vi "o3 Serial Data Recording & DECADEv3.1_test.vi"() -> ()   [LabVIEW 2014]
uses:
  <vilib>/Platform/TimedLoop/XDataNode/timing_clust.ctl
  <vilib>/Platform/TimedLoop/XDataNode/nitl_modes.ctl
  <vilib>/Platform/TimedLoop/XDataNode/wakeup.ctl
  C:/Program Files (x86)/National Instruments/LabVIEW 2014/examples/Data Communication/Network Streams/Simple Network Streams/support/Network Stream Command.ctl
  <vilib>/Utility/error.llb/whitespace.ctl
  <vilib>/Instr/_visa.llb/VISA Configure Serial Port (Instr).vi
  <vilib>/Utility/tcp.llb/UDP Multicast Write-Only Open.vi
  <vilib>/platform/TimedLoop/XDataNode/XDataNode.xnode
  <vilib>/Platform/TimedLoop/XDataNode/XDNodeRunTimeDep.lvlib
panel:
  out "Stop File Write":bool
  out "Default file name":string
  out "error out":errorcluster
  out "V6":bool
  in  "Clear Display\nErrors":bool
  out "Data Processing":bool
  out "Serial Visa Error":errorcluster
  out "SEPTIC TCP Error Out":errorcluster
  out "TCP packet\nSend to SEPTIC":bool
  in  "Time Stamp\nOffset":u32=1
  out "Data Array":string[](array[string])
  out "UDP packet \nstatus":bool
  out "UDP_Out_Error":errorcluster
  out "FISH TCP Error Out":errorcluster
  out "TCP packet\nSend to FISH":bool
  out "TCP Binary Packet":string
  out "Scan from String Error Counter\nfrom process loop":i32
  out "Read Error Counter\nfrom process loop":i32
  in  "milliseconds to wait":u32=330
  in  "ID":string="±"
  in  "VISA resource name":refnum<visa-resource-name>="ASRL6::INSTR"
  out "Data In Array":string[](array[string])
  out "UDP_ASCII_Out":string
  out "UDP_Pack_num":u32
  out "Flight Number":string
  in  "aux":string="0"
  in  "inlet_overq_mfm":string="0"
  in  "acs2653pc_hdd":string="0"
  in  "LabviewVIclient vn":string="0"
  in  "ue9LJ temp":u16
  in  "PTP Sync":string="0"
  out "Data String":string
  out "Internal packet":string[](array[string])
  out "RAW DATA":string
  in  "stop":bool
  out "Number of Send & Read Error\nfrom Acquire Loop":i32
  out "Command In":string
  # "o3_conc"
  # "Bench_temp"
  # "pressure"
  # "cell_a_nt"
  # "cell_b_int"
  # "flow_a"
  # "flow_b"
  # "lamp_temp"
  # "flags"
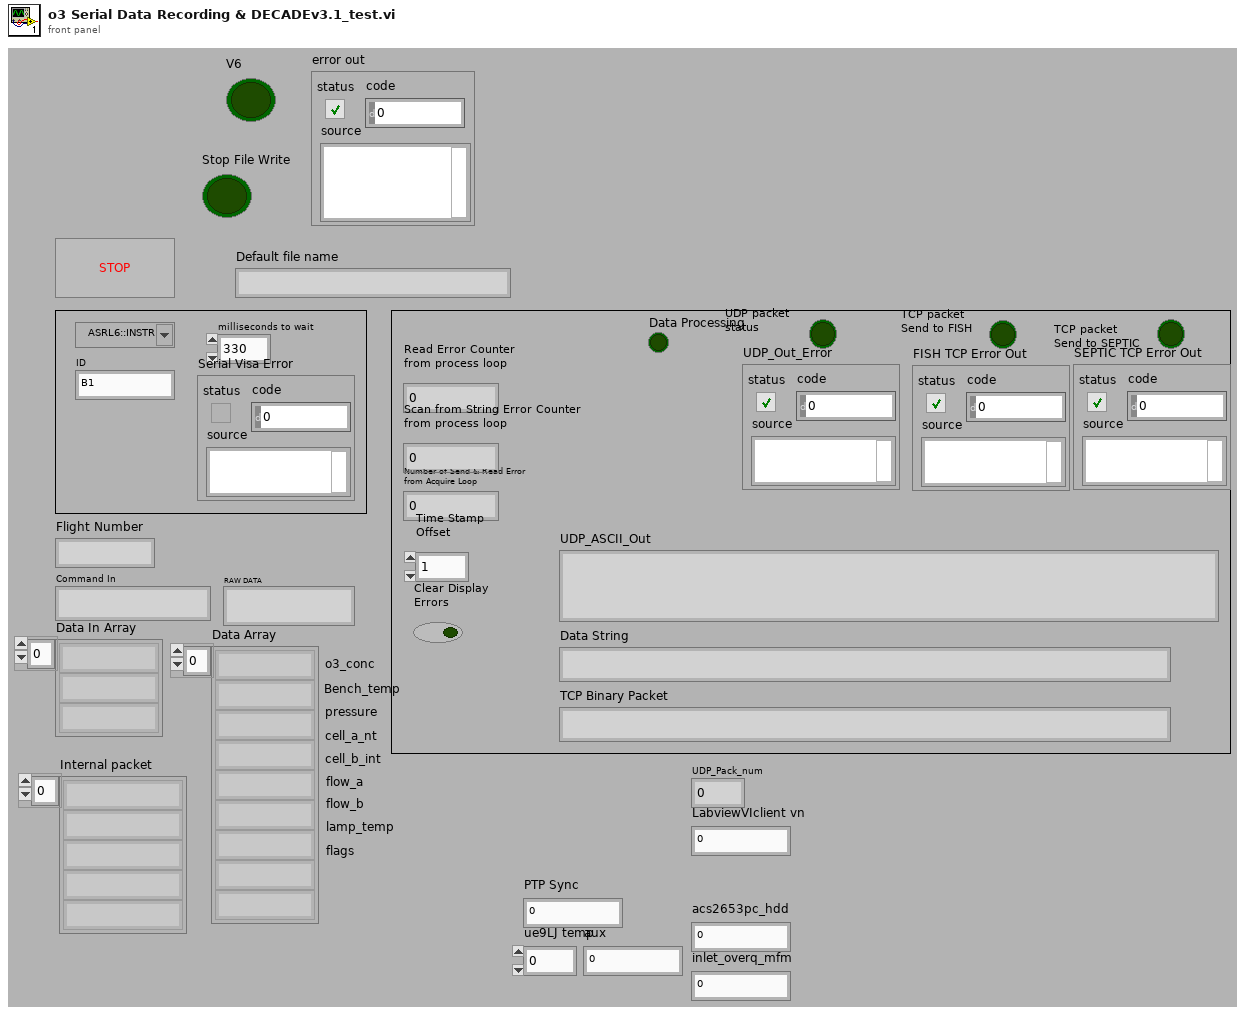
[diagram p1: front panel]
types:
  T1 = typedef "XDNodeRunTimeDep.lvlib/timing_clust.ctl" = cluster{"Expected End [f-1]":u64, "Actual End [f-1]":u64, "Finished Late? [f-1]":bool, "Expected End [i-1]":u64, "Actual End [i-1]":u64, "Finished Late? [i-1]":bool, "Expected Start [i]":u64, "Actual Start [i]":u64, "Expected Start [f]":u64, "Actual Start [f]":u64, "Source Name":string, "Structure Name":string, "Period":i64, "Deadline":i64, "Offset":i64, "Start":i64, "Priority":i32, "Timeout":i32, "Mode":T2, "Wakeup Reason":T3, "Error":errorcluster, "Source Type":string, "Secondary Source Type":string, "Global End Time":u64, "Global Start Time":u64, "Frame Duration":u64, "Iteration Duration":u64, "Assigned CPU":i32, "I/O Scan Engine Mode":u32}
  T2 = typedef "XDNodeRunTimeDep.lvlib/nitl_modes.ctl" = enum32{"No Change", "Process missed periods, maintain original phase", "Discard missed periods, maintain original phase", "Process missed periods, ignore original phase", "Discard missed periods, ignore original phase"}
  T3 = typedef "XDNodeRunTimeDep.lvlib/wakeup.ctl" = enum32{"Normal", "Aborted", "Asynchronous wakeup", "Timing source error", "Timed loop error", "Timeout"}
  T4 = typedef "Network Stream Command.ctl" = cluster{"Message":string, "Message Data":variant}
  T5 = enum16{"open", "replace", "create", "open or create", "replace or create", "replace or create with confirmation"}
  T6 = typedef "whitespace.ctl" = u16
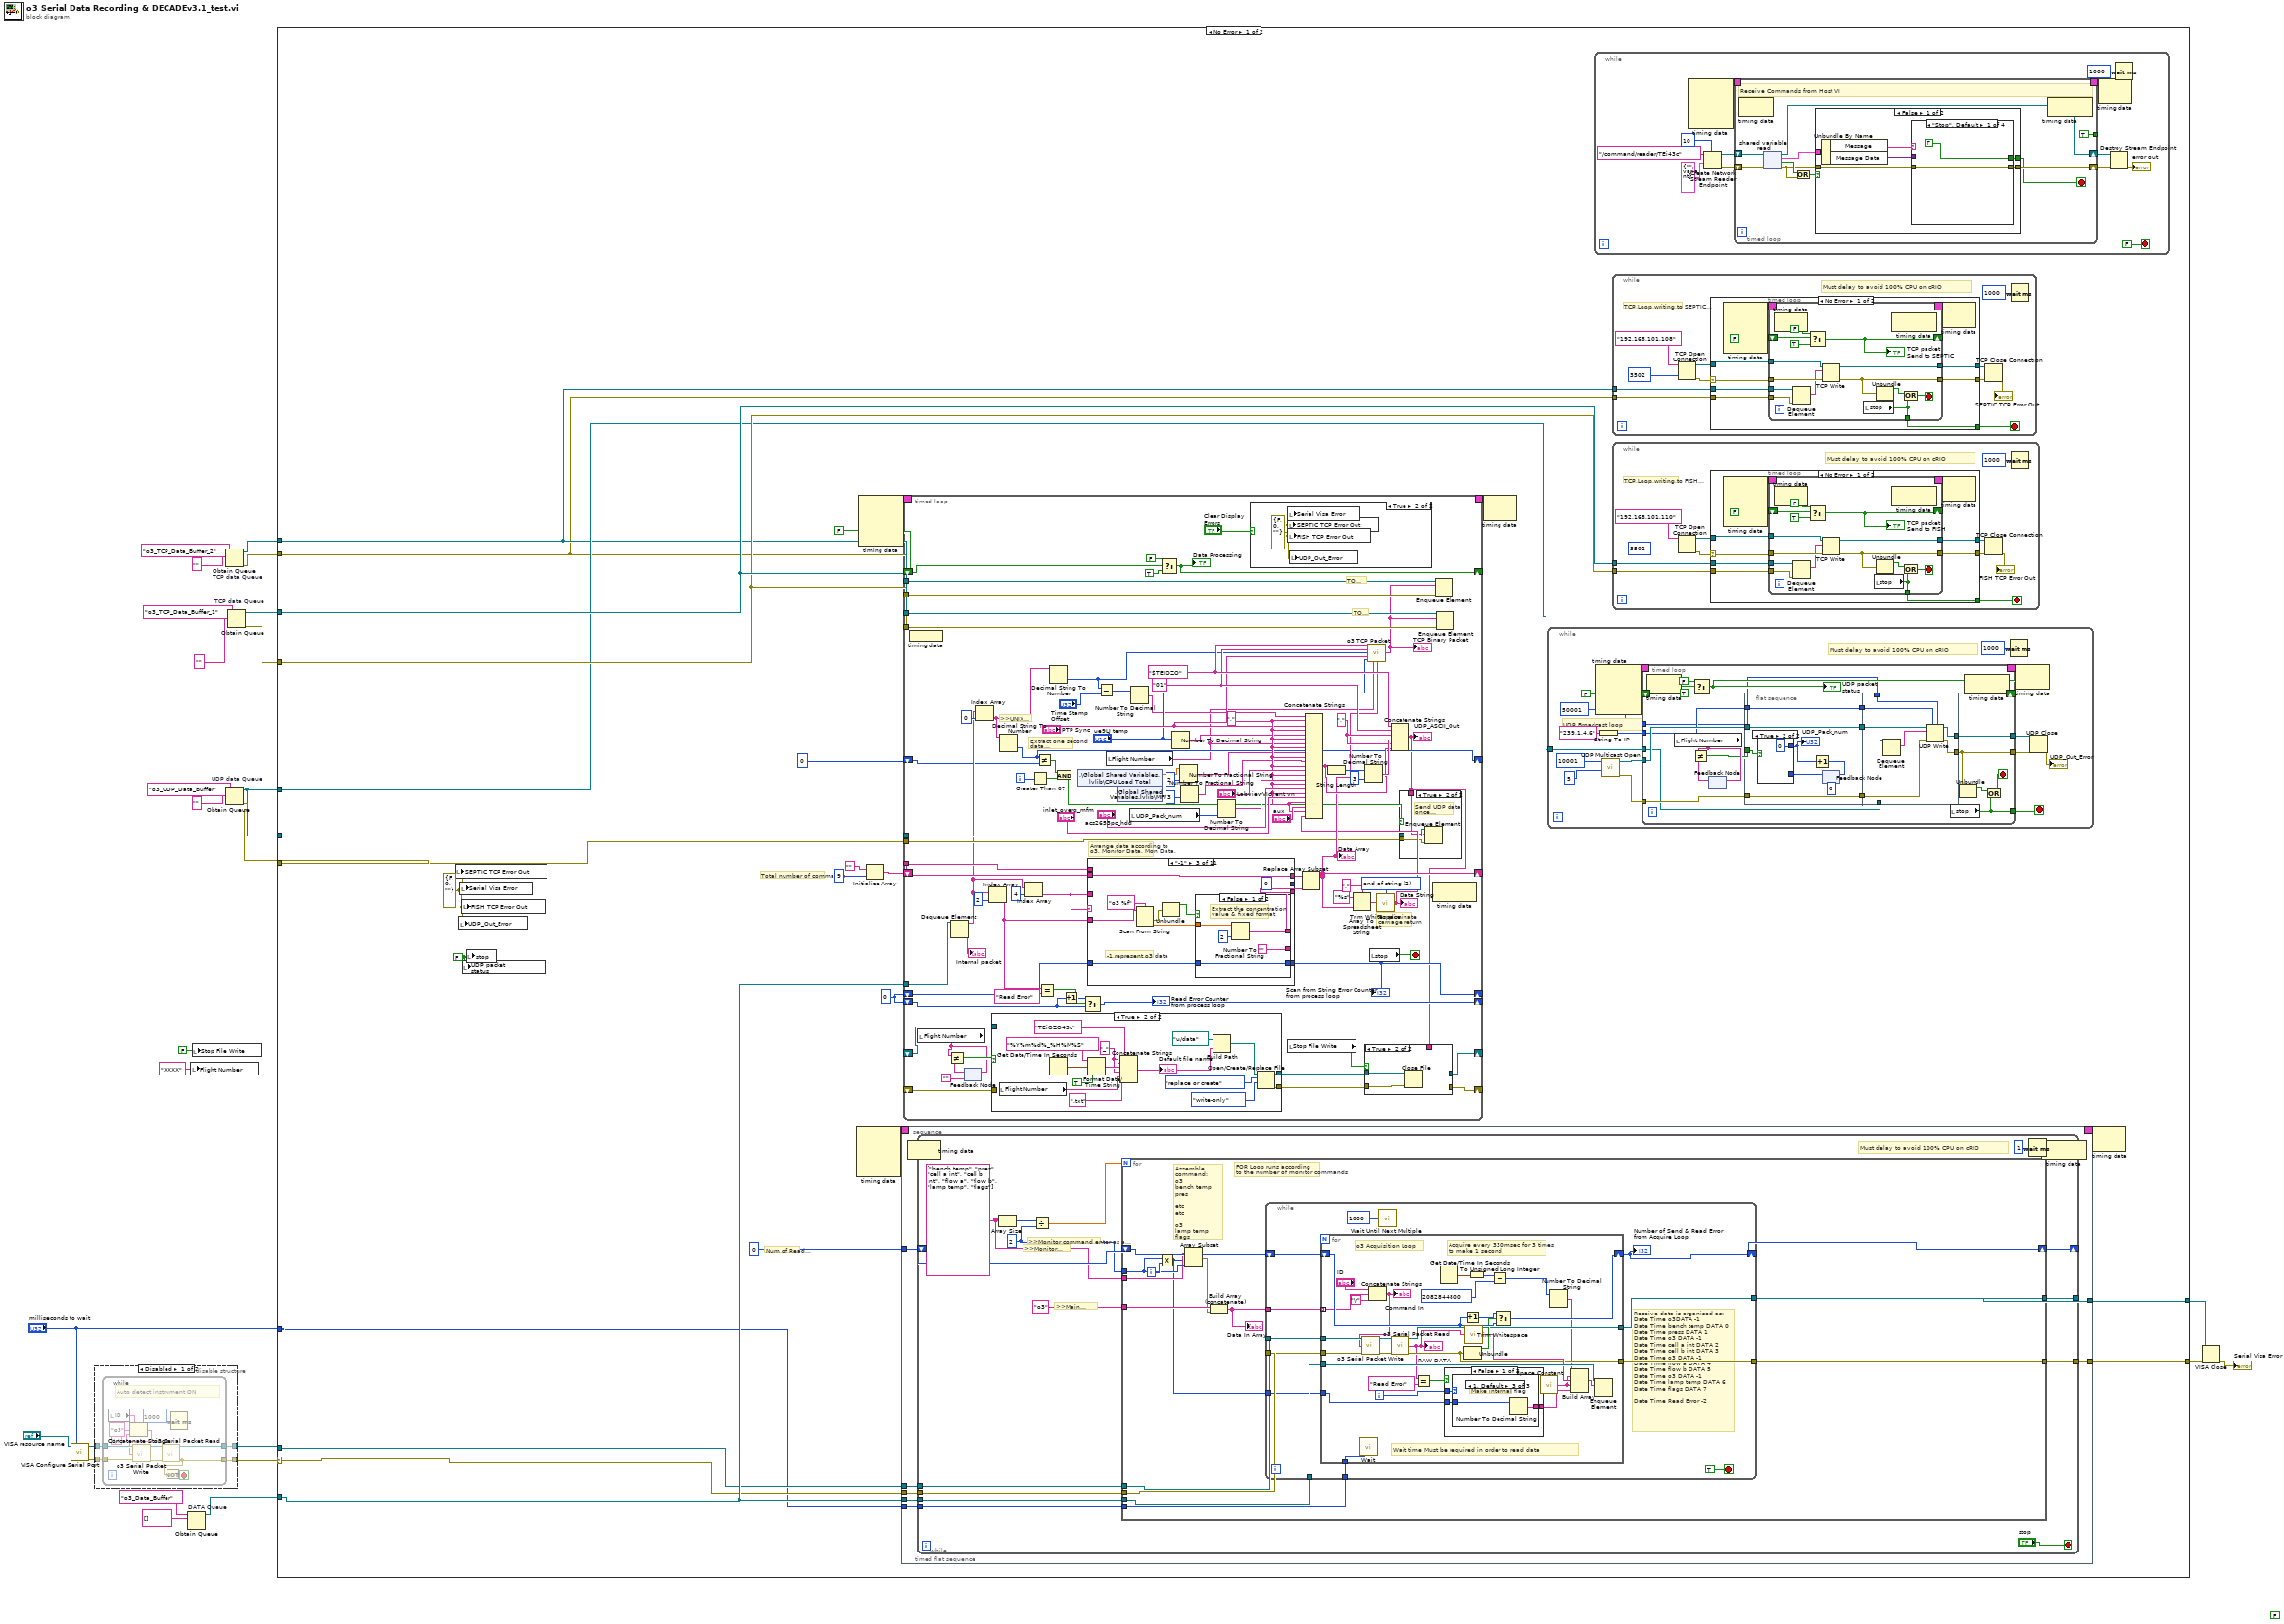
[diagram p0: block diagram]
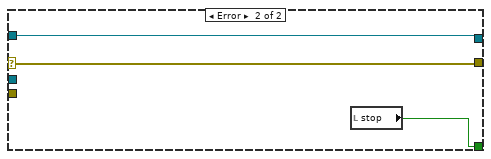
[diagram p3: hidden frame]
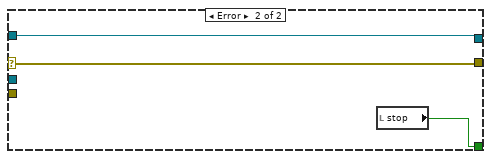
[diagram p4: hidden frame]
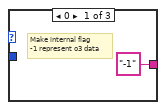
[diagram p5: hidden frame]
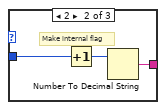
[diagram p6: hidden frame]
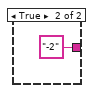
[diagram p7: hidden frame]
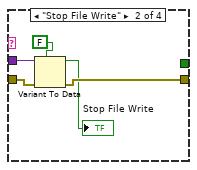
[diagram p8: hidden frame]
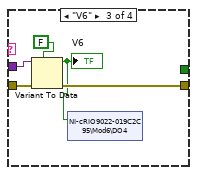
[diagram p9: hidden frame]
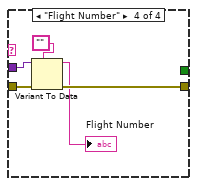
[diagram p10: hidden frame]
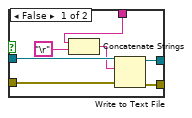
[diagram p14: hidden frame]
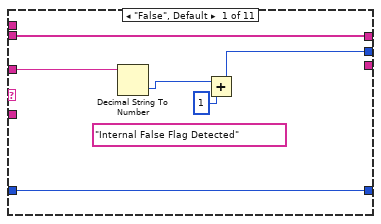
[diagram p17: hidden frame]
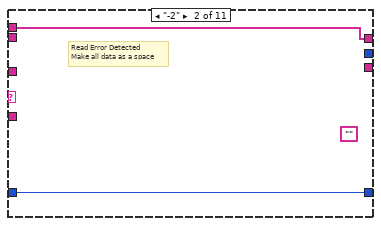
[diagram p18: hidden frame]
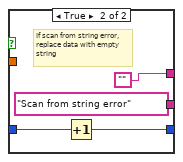
[diagram p19: hidden frame]
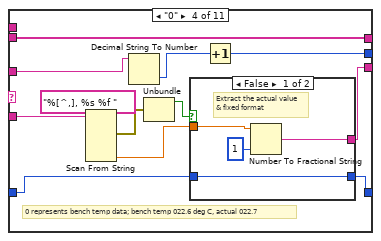
[diagram p20: hidden frame]
diagram:
  (unwired) FALSE
  n1 = call-poly "VISA Configure Serial Port"("VISA resource name"="VISA resource name", "timeout (10sec)"="milliseconds to wait") -> ("VISA resource name out"=w8:refnum<visa-resource-name>, "error out"=w7:errorcluster)  [unwired: 12 in]
  n2 = disable-structure shown="Disabled" {
    disable-tunnel: [w30 _] -> w10
    disable-tunnel: [w29 _] -> w9
    disable-tunnel: w8 -> [w28 _]
    disable-tunnel: w7 -> [w27 _]
    frame Disabled {
      n3 = while {
        tunnel: [w40] -> w30
        tunnel: [w39] -> w29
        tunnel: w28 -> [w38]
        tunnel: w27 -> [w37]
        stop <- w41 stop-if-true
        # "Auto detect instrument ON"
        n4 = local read "ID"() -> (w35:string)
        n5 = Concatenate Strings(w35, "o3" ("string"), "\r") -> (w32:string)
        n6 = call "o3 Serial Packet Write.vi"("VISA resource name In"=w38, "Data in"=w32, "error in (no error)"=w37) -> ("VISA resource name Out"=w36:refnum<visa-resource-name>, "error out"=w42:errorcluster)  [unwired: 11 in]
        n7 = call "o3 Serial Packet Read.vi"("VISA resource In"=w36, "error in"=w42) -> ("VISA resource Out"=w39:refnum<visa-resource-name>, "error out"=w40:errorcluster)  [unwired: 11 in, 1 out]
        n8 = Not(x=w40) -> (.not. x?=w41:bool)
        n9 = Wait (ms)(milliseconds to wait=u32 1000) -> ()  [unwired: 1 out]
      }
    }
    frame Enabled {
    }
  }
  n10 = Obtain Queue "DATA Queue"(name (unnamed)="o3_Data_Buffer", element data type=string[] []) -> (queue out=w24:refnum<queue>)  [unwired: 3 in, 2 out]
  n11 = local write "Flight Number"("XXXX" ("Flight Number")) -> ()
  n12 = local write "Stop File Write"(FALSE ("Stop File Write")) -> ()
  n13 = Obtain Queue "TCP data Queue"(name (unnamed)="o3_TCP_Data_Buffer_2", element data type="") -> (queue out=w13:refnum<queue>, error out=w12:errorcluster)  [unwired: 3 in, 1 out]
  n14 = Obtain Queue "UDP data Queue"(name (unnamed)="o3_UDP_Data_Buffer", element data type="") -> (queue out=w14:refnum<queue>, error out=w15:errorcluster)  [unwired: 3 in, 1 out]
  n15 = Obtain Queue "TCP data Queue"(name (unnamed)="o3_TCP_Data_Buffer_1", element data type="") -> (queue out=w19:refnum<queue>, error out=w18:errorcluster)  [unwired: 3 in, 1 out]
  n16 = case shown="No Error" w10 {
    selector: w10 -> [w52 w673]
    tunnel: [w68 w673] -> w21
    tunnel: [w67 w672] -> w22
    tunnel: w24 -> [w64 _]
    tunnel: w9 -> [w51 w672]
    tunnel: w19 -> [w57 _]
    tunnel: w18 -> [w56 _]
    tunnel: w14 -> [w55 _]
    tunnel: w15 -> [w54 _]
    tunnel: w14 -> [w53 _]
    tunnel: w13 -> [w49 _]
    tunnel: w12 -> [w48 _]
    tunnel: "milliseconds to wait" -> [w47 _]
    frame No Error {
      w45 = errorcluster {"status"=FALSE, "code"=0, "source"=""} ("UDP Error Out")
      w59 = 0
      w58 = FALSE ("stop")
      # "Num of Read Error"
      # "Total number of commands"
      n17 = local write "SEPTIC TCP Error Out"(w45) -> ()
      n18 = local write "UDP_Out_Error"(w45) -> ()
      n19 = local write "Serial Visa Error"(w45) -> ()
      n20 = local write "FISH TCP Error Out"(w45) -> ()
      n21 = local write "UDP packet \nstatus"(w58) -> ()
      n22 = local write "stop"(w58) -> ()
      n23 = node-c288() -> (w44:T1)  [unwired: 4 in]
      n24 = node-c288() -> (w66:T1)  [unwired: 4 in]
      n25 = Initialize Array("", 9) -> (w60:string[])
      n26 = timed-sequence {
        timing: w44 -> [_]
        timing-out: [_] -> w43
        tunnel: [w159] -> w68
        tunnel: [w158] -> w67
        tunnel: w64 -> [w157]
        tunnel: 0 -> [w156]
        tunnel: w52 -> [w155]
        tunnel: w51 -> [w154]
        tunnel: w47 -> [w153]
        n27 = timed-flat-sequence {
          tunnel: [w166] -> w159
          tunnel: [w165] -> w158
          tunnel: w157 -> [w164]
          tunnel: w156 -> [w163]
          tunnel: w155 -> [w162]
          tunnel: w154 -> [w161]
          tunnel: w153 -> [w160]
          n28 = node-c288() -> ()  [unwired: 1 in, 1 out]
          n29 = while {
            tunnel: [w170] -> w166
            tunnel: w161 -> [w181]
            tunnel: w162 -> [w180]
            tunnel: [w179] -> w165
            tunnel: w164 -> [w178]
            shift-right: [w176] -> _
            shift-left: w163 -> [w177]
            tunnel: w160 -> [w168]
            stop <- "stop" stop-if-true
            w171 = 2
            w173 = string[] ["bench temp", "pres", "cell a int", "cell b int", "flow a", "flow b", "lamp temp", "flags"]
            # "Must delay to avoid 100% CPU on cRIO"
            # ">>Monitor command enter as a pair>>"
            # ">>Main commands>>"
            # ">>Monitor Command>>"
            n30 = Array Size(array=w173) -> (size(s)=w174:i32)
            n31 = Divide(x=w174, y=w171) -> (x/y=w172:dbl)
            n32 = for {
              N: w172 -> [_]
              tunnel: w181 -> [w189]
              tunnel: w180 -> [w188]
              tunnel: [w196] -> w170
              shift-right: [w194] -> w176
              shift-left: w177 -> [w195]
              tunnel: [w193] -> w179
              tunnel: w178 -> [w192]
              tunnel: w173 -> [w185]
              tunnel: "o3" -> [w190]
              tunnel: w171 -> [w186]
              tunnel: w168 -> [w182]
              i -> [w187]
              # "FOR Loop runs according\nto the number of monitor commands"
              # "Assemble command:\no3\nbench temp\npres\n\netc\netc\n\no3\nlamp temp\nflags"
              n33 = Multiply(x=w186, y=w187) -> (x*y=w183:i32)
              n34 = Array Subset(array=w185, index=w183, length=w186) -> (w184:string[])
              n35 = Build Array (concatenate)(w190, w184) -> (w191:string[])
              "Data In Array" <- w191
              n36 = while {
                tunnel: [w208] -> w196
                tunnel: w191 -> [w206]
                tunnel: [w204] -> w193
                tunnel: w192 -> [w203]
                tunnel: w188 -> [w202]
                tunnel: w189 -> [w201]
                tunnel: w183 -> [w200]
                shift-right: [w205] -> w194
                shift-left: w195 -> [w207]
                tunnel: w182 -> [w197]
                stop <- TRUE stop-if-true
                # "Receive data is organised as:\nDate Time o3DATA -1\nDate Time bench temp DATA 0\nDate Time press DATA 1\nDate Time o3 DATA -1\nDate Time cell a int DATA 2\nDate Time cell b int DATA 3\nDate Time o3 DATA -1\nDate Time flow a DATA 4\nDate Time flow b DATA 5\nDate Time o3 DATA -1\nDate Time lamp temp DATA 6\nDate Time flags DATA 7\n\nDate Time Read Error -2"
                n37 = for {
                  tunnel: w202 -> [w225]
                  tunnel: [w226] -> w208
                  tunnel: w206 -> [w223] mode=indexing
                  tunnel: [w227] -> w204
                  tunnel: w203 -> [w233]
                  tunnel: w201 -> [w228]
                  tunnel: w200 -> [w222]
                  shift-right: [w237] -> w205
                  shift-left: w207 -> [w238]
                  tunnel: w197 -> [w211]
                  i -> [w215]
                  # "Wait time Must be required in order to read data"
                  # "Acquire every 330msec for 3 times\nto make 1 second"
                  # "o3 Acquisition Loop"
                  n38 = call "Wait"("Count(mSec)"=w211) -> ()  [unwired: 1 out]
                  n39 = Concatenate Strings("ID", w223, "\r") -> (w221:string)
                  "Command In" <- w221
                  n40 = call "o3 Serial Packet Write.vi"("VISA resource name In"=w228, "Data in"=w221, "error in (no error)"=w225) -> ("VISA resource name Out"=w230:refnum<visa-resource-name>, "error out"=w229:errorcluster)  [unwired: 11 in]
                  n41 = call "o3 Serial Packet Read.vi"("VISA resource In"=w230, "error in"=w229) -> ("VISA resource Out"=w227:refnum<visa-resource-name>, "Data Out"=w218:string, "error out"=w226:errorcluster)  [unwired: 11 in]
                  "RAW DATA" <- w218
                  n42 = Equal?(x=w218, y="Read Error") -> (x = y?=w216:bool)
                  n43 = Get Date/Time In Seconds() -> (seconds since 1Jan1904=w210:timestamp)
                  n44 = case shown="False" w216 {
                    tunnel: [w241 "-2"] -> w231
                    tunnel: w215 -> [w240 _]
                    tunnel: w222 -> [w239 _]
                    frame False {
                      n45 = case shown="1, Default" w240 {
                        tunnel: ["-1" w245 w247] -> w241
                        tunnel: w239 -> [_ w243 w246]
                        frame 0 {
                          # "Make internal flag\n-1 represent o3 data"
                        }
                        frame 2 {
                          # "Make internal flag"
                          n46 = Increment(x=w243) -> (x+1=w244:i32)
                          n47 = Number To Decimal String(number=w244) -> (decimal integer string=w245:string)  [unwired: 1 in]
                        }
                        frame 1, Default {
                          # "Make internal flag"
                          n48 = Number To Decimal String(number=w246) -> (decimal integer string=w247:string)  [unwired: 1 in]
                        }
                      }
                    }
                    frame True {
                    }
                  }
                  n49 = Increment(x=w238) -> (x+1=w234:i32)
                  n50 = Unbundle(w226) -> ("status"=w235:bool)  [unwired: 2 out]
                  n51 = call <vilib>:"Trim Whitespace.vi"("string"=w218) -> ("trimmed string"=w232:string)  [unwired: 1 in]
                  n52 = To Unsigned Long Integer(number=w210) -> (unsigned 32bit integer=w214:u32)
                  n53 = Subtract(x=w214, y=u32 2082844800) -> (x-y=w209:u32)
                  n54 = Select(t=w234, s=w235, f=w238) -> (s? t:f=w237:i32)
                  n55 = call <vilib>:"Space Constant.vi"() -> ("String"=w219:string)
                  n56 = Number To Decimal String(number=w209) -> (decimal integer string=w212:string)  [unwired: 1 in]
                  n57 = Build Array(w212, w219, w232, w219, w231) -> (w220:string[])
                  n58 = Enqueue Element(queue=w233, element=w220) -> ()  [unwired: 2 in, 3 out]
                }
                "Number of Send & Read Error\nfrom Acquire Loop" <- w205
                n59 = call "Wait Until Next Multiple"("Count(mSec)"=u32 1000) -> ()  [unwired: 1 out]
              }
            }
            n60 = Wait (ms)(milliseconds to wait=u32 1) -> ()  [unwired: 1 out]
          }
          n61 = node-c288() -> ()  [unwired: 1 in, 1 out]
        }
      }
      n62 = timed-loop {
        timing: w66 -> [_]
        timing-out: [_] -> w65
        tunnel: w64 -> [w446]
        shift-right: [w407] -> _
        shift-left: w60 -> [w430]
        shift-right: [w418] -> _
        shift-left: w59 -> [w415]
        tunnel: w60 -> [w417]
        shift-right: [w413] -> _
        shift-left: w59 -> [w414]
        tunnel: w57 -> [w406]
        tunnel: w56 -> [w405]
        tunnel: w55 -> [w403]
        tunnel: w54 -> [w402]
        shift-right: [w394] -> _
        shift-left: 0 -> [w397]
        tunnel: w49 -> [w392]
        tunnel: w48 -> [w391]
        shift-right: [w382] -> _
        shift-left: FALSE -> [w385]
        shift-right: [w379] -> _
        shift-left: _ -> [w370]
        shift-right: [w368] -> _
        shift-left: _ -> [w369]
        i -> [w395]
        stop <- w444 stop-if-true
        w423 = T6 2 items=["both", "start of string", "end of string"] ("location (both)")
        w436 = ","
        w410 = "01"
        w432 = ","
        w411 = "$TEIOZO"
        # "TO SEPTIC"
        # "TO FISH"
        # "Extract one second data\nfor UDP sending"
        # "Arrange data according to\no3, Monitor Data, Mon Data,"
        # "To eliminate\ncarriage return"
        # ">>UNIX TIME>>"
        n63 = node-c288() -> ()  [unwired: 1 in]
        n64 = local read "Flight Number"() -> (w373:string)
        n65 = Dequeue Element(queue=w446) -> (element=w400:string[])  [unwired: 2 in, 3 out]
        "Internal packet" <- w400
        n66 = feedback #1("" ("Flight Number")) -> (w375:string)
        n67 = Not Equal?(x=w373, y=w375) -> (x != y?=w374:bool)
        n68 = feedback-in #1(w373) -> ()
        n69 = Index Array(array=w400, index=0) -> (element=w399:string)
        n70 = Index Array(array=w400, index=2) -> (element=w421:string)
        n71 = case shown="True" w374 {
          tunnel: [w448 w450] -> w372
          tunnel: [w447 w449] -> w371
          tunnel: w370 -> [w448 _]
          tunnel: w369 -> [w447 _]
          frame False {
          }
          frame True {
            w457 = "_" ("string")
            n72 = local read "Flight Number"() -> (w463:string)
            n73 = Get Date/Time In Seconds() -> (seconds since 1Jan1904=w458:timestamp)
            n74 = Format Date/Time String(time format string (%c)="%Y%m%d%_%H%M%S", seconds (now)=w458, UTC format=TRUE) -> (date/time string=w461:string)
            n75 = Concatenate Strings("TEiOZO43c" ("string"), w457, w461, w457, w463, ".txt" ("string")) -> (w455:string)
            "Default file name" <- w455
            n76 = Build Path(base path=path "u:/data", name or relative path=w455) -> (appended path=w451:path)
            n77 = Open/Create/Replace File(file path (use dialog)=w451, operation (0:open)=T5."replace or create", access (0:read/write)=enum16{"read/write", "read-only", "write-only"}."write-only") -> (refnum out=w450:refnum<file>, error out=w449:errorcluster)  [unwired: 3 in, 1 out]
          }
        }
        n78 = Decimal String To Number(string=w399) -> (number=w394:i32)  [unwired: 2 in, 1 out]
        n79 = Index Array(array=w400, index=4) -> (element=w429:string)
        n80 = Greater Than 0?(x=w395) -> (x > 0?=w398:bool)
        n81 = Not Equal?(x=w394, y=w397) -> (x != y?=w396:bool)
        n82 = Equal?(x=w421, y="Read Error") -> (x = y?=w419:bool)
        n83 = Decimal String To Number(string=w399) -> (number=w388:i32)  [unwired: 2 in, 1 out]
        n84 = Compound Arithmetic op=AND(w396, w398) -> (w393:bool)
        n85 = Increment(x=w415) -> (x+1=w416:i32)
        n86 = shared-variable ".\\Global Shared Variables.lvlib\\CPU Load Total"() -> (w367:dbl)  [unwired: 1 in, 1 out]
        n87 = Select(t=w416, s=w419, f=w415) -> (s? t:f=w418:i32)
        "Read Error Counter\nfrom process loop" <- w418
        n88 = case shown="\"-1\"" w429 {
          tunnel: w429 -> [w481 _ _ w514 w533 w554 w575 w596 w617 w638 w659]
          tunnel: w430 -> [w482 _ w494 w515 w534 w555 w576 w597 w618 w639 w660]
          tunnel: w421 -> [_ _ w491 w510 w529 w551 w572 w593 w614 w635 w656]
          tunnel: [w482 w484 w494 w515 w534 w555 w576 w597 w618 w639 w660] -> w428
          tunnel: [w479 _ 0 ("index") w512 w531 w552 w573 w594 w615 w636 w657] -> w427
          tunnel: [_ _ w489 w508 w527 w550 w571 w592 w613 w634 w651] -> w426
          tunnel: w417 -> [_ w484 _ _ _ _ _ _ _ _ _]
          tunnel: w414 -> [w477 w483 w486 w505 w524 w545 w566 w587 w608 w629 w650]
          tunnel: [w477 w483 w485 w504 w523 w544 w565 w586 w607 w628 w649] -> w413
          frame "False", Default {
            (unwired) "Internal False Flag Detected"
            n89 = Decimal String To Number(string=w481) -> (number=w478:i32)  [unwired: 2 in, 1 out]
            n90 = Add(x=w478, y=1) -> (x+y=w479:i32)
          }
          frame "-2" {
            (unwired) ""
            # "Read Error Detected\nMake all data as a space"
          }
          frame "-1" {
            # "-1 represent o3 data"
            n91 = Scan From String(format string="o3 %f", input string=w491) -> (error out=w488:errorcluster, output 1=w490:dbl)  [unwired: 3 in, 2 out]
            n92 = Unbundle(w488) -> ("status"=w487:bool)  [unwired: 2 out]
            n93 = case shown="False" w487 {
              tunnel: w490 -> [w499 _]
              tunnel: [w498 ""] -> w489
              tunnel: w486 -> [w497 w502]
              tunnel: [w497 w501] -> w485
              tunnel: ["" "Scan from string error"] -> _
              frame False {
                # "Extract the concentration\nvalue & fixed format"
                n94 = Number To Fractional String(number=w499, precision (6)=i16 2) -> (F-format string=w498:string)  [unwired: 2 in]
              }
              frame True {
                # "If scan from string error,\nreplace data with empty\nstring"
                n95 = Increment(x=w502) -> (x+1=w501:i32)
              }
            }
          }
          frame "0" {
            # "0 represents bench temp data; bench temp 022.6 deg C, actual 022.7"
            n96 = Scan From String(format string="%[^,], %s %f ", input string=w510) -> (error out=w507:errorcluster, output 3=w509:dbl)  [unwired: 7 in, 2 out]
            n97 = Decimal String To Number(string=w514) -> (number=w513:i32)  [unwired: 2 in, 1 out]
            n98 = Unbundle(w507) -> ("status"=w506:bool)  [unwired: 2 out]
            n99 = case shown="False" w506 {
              tunnel: w509 -> [w519 _]
              tunnel: [w518 ""] -> w508
              tunnel: w505 -> [w517 w521]
              tunnel: [w517 w520] -> w504
              frame False {
                # "Extract the actual value\n& fixed format"
                n100 = Number To Fractional String(number=w519, precision (6)=i16 1) -> (F-format string=w518:string)  [unwired: 2 in]
              }
              frame True {
                (unwired) "Scan from string error"
                # "If scan from string error,\nreplace data with empty\nstring"
                n101 = Increment(x=w521) -> (x+1=w520:i32)
              }
            }
            n102 = Increment(x=w513) -> (x+1=w512:i32)
          }
          frame "1" {
            # "1 represents pres data; pres 725.3 mmHg, actual 725.4"
            n103 = Scan From String(format string="%[^,], %s %f ", input string=w529) -> (error out=w526:errorcluster, output 3=w528:dbl)  [unwired: 7 in, 2 out]
            n104 = Decimal String To Number(string=w533) -> (number=w532:i32)  [unwired: 2 in, 1 out]
            n105 = Unbundle(w526) -> ("status"=w525:bool)  [unwired: 2 out]
            n106 = case shown="False" w525 {
              tunnel: w528 -> [w539 _]
              tunnel: [w538 ""] -> w527
              tunnel: w524 -> [w537 w542]
              tunnel: [w537 w541] -> w523
              tunnel: ["" "Scan from string error"] -> _
              frame False {
                # "Extract the actual value\n& fixed format"
                n107 = Number To Fractional String(number=w539, precision (6)=i16 1) -> (F-format string=w538:string)  [unwired: 2 in]
              }
              frame True {
                # "If scan from string error,\nreplace data with empty\nstring"
                n108 = Increment(x=w542) -> (x+1=w541:i32)
              }
            }
            n109 = Increment(x=w532) -> (x+1=w531:i32)
          }
          frame "2" {
            # "2 represents cell a int data; cell a int 63246 Hz"
            n110 = Scan From String(format string="cell a int %d", input string=w551) -> (error out=w547:errorcluster, output 1=w548:i32)  [unwired: 3 in, 2 out]
            n111 = Decimal String To Number(string=w554) -> (number=w553:i32)  [unwired: 2 in, 1 out]
            n112 = Unbundle(w547) -> ("status"=w546:bool)  [unwired: 2 out]
            n113 = case shown="False" w546 {
              tunnel: [w560 ""] -> w550
              tunnel: w548 -> [w559 _]
              tunnel: w545 -> [w558 w563]
              tunnel: [w558 w562] -> w544
              tunnel: ["" "Scan from string error"] -> _
              frame False {
                # "Extract the actual value\n& fixed format"
                n114 = Number To Fractional String(number=w559, precision (6)=i16 0) -> (F-format string=w560:string)  [unwired: 2 in]
              }
              frame True {
                # "If scan from string error,\nreplace data with empty\nstring"
                n115 = Increment(x=w563) -> (x+1=w562:i32)
              }
            }
            n116 = Increment(x=w553) -> (x+1=w552:i32)
          }
          frame "3" {
            # "3 represents cell b int data; cell b int 63246 Hz"
            n117 = Scan From String(format string="cell b int %d", input string=w572) -> (error out=w568:errorcluster, output 1=w569:i32)  [unwired: 3 in, 2 out]
            n118 = Decimal String To Number(string=w575) -> (number=w574:i32)  [unwired: 2 in, 1 out]
            n119 = Unbundle(w568) -> ("status"=w567:bool)  [unwired: 2 out]
            n120 = case shown="False" w567 {
              tunnel: [w581 ""] -> w571
              tunnel: w569 -> [w580 _]
              tunnel: w566 -> [w579 w584]
              tunnel: [w579 w583] -> w565
              tunnel: ["" "Scan from string error"] -> _
              frame False {
                # "Extract the actual value\n& fixed format"
                n121 = Number To Fractional String(number=w580, precision (6)=i16 0) -> (F-format string=w581:string)  [unwired: 2 in]
              }
              frame True {
                # "If scan from string error,\nreplace data with empty\nstring"
                n122 = Increment(x=w584) -> (x+1=w583:i32)
              }
            }
            n123 = Increment(x=w574) -> (x+1=w573:i32)
          }
          frame "4" {
            # "4 represents flow a data; flow a 0.696 l/m"
            n124 = Scan From String(format string="flow a %f", input string=w593) -> (error out=w589:errorcluster, output 1=w590:dbl)  [unwired: 3 in, 2 out]
            n125 = Decimal String To Number(string=w596) -> (number=w595:i32)  [unwired: 2 in, 1 out]
            n126 = Unbundle(w589) -> ("status"=w588:bool)  [unwired: 2 out]
            n127 = case shown="False" w588 {
              tunnel: [w602 ""] -> w592
              tunnel: w590 -> [w601 _]
              tunnel: w587 -> [w600 w605]
              tunnel: [w600 w604] -> w586
              tunnel: ["" "Scan from string error"] -> _
              frame False {
                # "Extract the actual value\n& fixed format"
                n128 = Number To Fractional String(number=w601, precision (6)=i16 3) -> (F-format string=w602:string)  [unwired: 2 in]
              }
              frame True {
                # "If scan from string error,\nreplace data with empty\nstring"
                n129 = Increment(x=w605) -> (x+1=w604:i32)
              }
            }
            n130 = Increment(x=w595) -> (x+1=w594:i32)
          }
          frame "5" {
            # "5 represents flow b data; flow b 0.696 l/m"
            n131 = Scan From String(format string="flow b %f", input string=w614) -> (error out=w610:errorcluster, output 1=w611:dbl)  [unwired: 3 in, 2 out]
            n132 = Decimal String To Number(string=w617) -> (number=w616:i32)  [unwired: 2 in, 1 out]
            n133 = Unbundle(w610) -> ("status"=w609:bool)  [unwired: 2 out]
            n134 = case shown="False" w609 {
              tunnel: [w623 ""] -> w613
              tunnel: w611 -> [w622 _]
              tunnel: w608 -> [w621 w626]
              tunnel: [w621 w625] -> w607
              tunnel: ["" "Scan from string error"] -> _
              frame False {
                # "Extract the actual value\n& fixed format"
                n135 = Number To Fractional String(number=w622, precision (6)=i16 3) -> (F-format string=w623:string)  [unwired: 2 in]
              }
              frame True {
                # "If scan from string error,\nreplace data with empty\nstring"
                n136 = Increment(x=w626) -> (x+1=w625:i32)
              }
            }
            n137 = Increment(x=w616) -> (x+1=w615:i32)
          }
          frame "6" {
            # "6 represents lamp temp data; lamp temp 056.1 deg C"
            n138 = Scan From String(format string="lamp temp %f", input string=w635) -> (error out=w631:errorcluster, output 1=w632:dbl)  [unwired: 3 in, 2 out]
            n139 = Decimal String To Number(string=w638) -> (number=w637:i32)  [unwired: 2 in, 1 out]
            n140 = Unbundle(w631) -> ("status"=w630:bool)  [unwired: 2 out]
            n141 = case shown="False" w630 {
              tunnel: [w644 ""] -> w634
              tunnel: w632 -> [w643 _]
              tunnel: w629 -> [w642 w647]
              tunnel: [w642 w646] -> w628
              tunnel: ["" "Scan from string error"] -> _
              frame False {
                # "Extract the actual value\n& fixed format"
                n142 = Number To Fractional String(number=w643, precision (6)=i16 1) -> (F-format string=w644:string)  [unwired: 2 in]
              }
              frame True {
                # "If scan from string error,\nreplace data with empty\nstring"
                n143 = Increment(x=w647) -> (x+1=w646:i32)
              }
            }
            n144 = Increment(x=w637) -> (x+1=w636:i32)
          }
          frame "7" {
            # "7 represents flags data; flags 1c100000"
            n145 = Scan From String(format string="flags %s", input string=w656) -> (error out=w654:errorcluster, output 1=w652:string)  [unwired: 3 in, 2 out]
            n146 = Decimal String To Number(string=w659) -> (number=w658:i32)  [unwired: 2 in, 1 out]
            n147 = Unbundle(w654) -> ("status"=w653:bool)  [unwired: 2 out]
            n148 = case shown="False" w653 {
              tunnel: w652 -> [w663 _]
              tunnel: [w663 ""] -> w651
              tunnel: w650 -> [w662 w666]
              tunnel: [w662 w665] -> w649
              tunnel: ["" "Scan from string error"] -> _
              frame False {
                # "Extract the actual value\n& fixed format"
              }
              frame True {
                # "If scan from string error,\nreplace data with empty\nstring"
                n149 = Increment(x=w666) -> (x+1=w665:i32)
              }
            }
            n150 = Increment(x=w658) -> (x+1=w657:i32)
          }
        }
        "Scan from String Error Counter\nfrom process loop" <- w413
        n151 = Subtract(x=w388, y="Time Stamp\nOffset") -> (x-y=w389:u32)
        n152 = local read "Flight Number"() -> (w377:string)
        n153 = shared-variable ".\\Global Shared Variables.lvlib\\MFM"() -> (w366:dbl)  [unwired: 1 in, 1 out]
        n154 = local read "UDP_Pack_num"() -> (w441:u32)
        n155 = Number To Decimal String(number=w389) -> (decimal integer string=w386:string)  [unwired: 1 in]
        n156 = Select(t=FALSE, s=w385, f=TRUE) -> (s? t:f=w382:bool)
        "Data Processing" <- w382
        n157 = Number To Decimal String(number="ue9LJ temp") -> (decimal integer string=w412:string)  [unwired: 1 in]
        n158 = Number To Fractional String(number=w367, precision (6)=i16 2) -> (F-format string=w364:string)  [unwired: 2 in]
        n159 = Number To Fractional String(number=w366, precision (6)=i16 3) -> (F-format string=w362:string)  [unwired: 2 in]
        n160 = Number To Decimal String(number=w441) -> (decimal integer string=w440:string)  [unwired: 1 in]
        n161 = case shown="True" "Clear Display\nErrors" {
          frame False {
          }
          frame True {
            w473 = errorcluster {"status"=FALSE, "code"=0, "source"=""} ("UDP Error Out")
            n162 = local write "SEPTIC TCP Error Out"(w473) -> ()
            n163 = local write "Serial Visa Error"(w473) -> ()
            n164 = local write "FISH TCP Error Out"(w473) -> ()
            n165 = local write "UDP_Out_Error"(w473) -> ()
          }
        }
        n166 = local read "Stop File Write"() -> (w378:bool)
        n167 = Replace Array Subset(array=w428, new element=w426, index=w427) -> (w407:string[])
        "Data Array" <- w407
        n168 = Array To Spreadsheet String(delimiter (Tab)=",", array=w407, 3:"%s" ("format string")) -> (spreadsheet string=w422:string)
        n169 = call "o3 TCP Packet.vi"("ID"=w411, "Version"=w410, "utc_time"=w388, "PTP Sync"="PTP Sync", "ue9LJ temp"="ue9LJ temp", "Flight Number"=w377, "Data Array"=w407) -> ("TCP Binary Packet"=w390:string)  [unwired: 8 in]
        "TCP Binary Packet" <- w390
        n170 = local read "stop"() -> (w444:bool)
        n171 = call <vilib>:"Trim Whitespace.vi"("string"=w422, "location (both)"=w423) -> ("trimmed string"=w404:string)
        "Data String" <- w404
        n172 = Concatenate Strings(w386, w436, "PTP Sync", w436, w412, w436, w377, w436, w364, w436, w362, w436, "LabviewVIclient vn", w436, w440, w436, "acs2653pc_hdd", w436, "inlet_overq_mfm", w436, "aux", w436, w404) -> (w431:string)
        n173 = String Length(string=w431) -> (length=w435:i32)
        n174 = Number To Decimal String(number=w435, width (-)=i16 3) -> (decimal integer string=w433:string)
        n175 = Concatenate Strings(w411, w410, w432, w433, w432, w431) -> (w380:string)
        "UDP_ASCII_Out" <- w380
        n176 = case shown="True" w378 {
          tunnel: w372 -> [w470 w472]
          tunnel: w371 -> [w469 w471]
          tunnel: [w466 _] -> w379
          tunnel: w380 -> [w465 _]
          tunnel: [w464 _] -> w368
          frame False {
            n177 = Concatenate Strings(w465, "\r") -> (w467:string)
            n178 = Write to Text File(file (use dialog)=w470, text=w467, error in=w469) -> (refnum out=w466:refnum<file>, error out=w464:errorcluster)  [unwired: 2 out]
          }
          frame True {
            n179 = Close File(refnum=w472, error in=w471) -> ()  [unwired: 2 out]
          }
        }
        n180 = case shown="True" w393 {
          tunnel: w403 -> [_ w476]
          tunnel: w402 -> [_ w475]
          tunnel: w380 -> [_ w474]
          frame False {
          }
          frame True {
            # "Send UDP data once\na second"
            n181 = Enqueue Element(queue=w476, element=w474, error in (no error)=w475) -> ()  [unwired: 1 in, 3 out]
          }
        }
        n182 = node-c288() -> ()  [unwired: 1 in, 1 out]
        n183 = Enqueue Element(queue=w392, element=w390, error in (no error)=w391) -> ()  [unwired: 1 in, 3 out]
        n184 = Enqueue Element(queue=w406, element=w390, error in (no error)=w405) -> ()  [unwired: 1 in, 3 out]
      }
      n185 = node-c288(w65) -> ()  [unwired: 1 out]
      n186 = while {
        tunnel: w53 -> [w305]
        stop <- w306 stop-if-true
        # "Must delay to avoid 100% CPU on cRIO"
        # "UDP Broadcast loop"
        n187 = node-c288() -> (w308:T1)  [unwired: 4 in]
        n188 = String To IP(1:"239.1.4.6" ("name")) -> (0:w310:u32)
        n189 = call-poly <vilib>:"UDP Multicast Open.vi"("time-to-live (1)"=u16 5, "port"=u16 10001) -> ("error out"=w318:errorcluster, "connection ID"=w319:refnum<k16>)  [unwired: 8 in]
        n190 = timed-loop {
          tunnel: w319 -> [w339]
          tunnel: w318 -> [w338]
          tunnel: [w325] -> w314
          shift-right: [w328] -> _
          shift-left: FALSE -> [w331]
          tunnel: [w323] -> w312
          tunnel: w310 -> [w327]
          tunnel: u16 50001 ("port or service name") -> [w326]
          timing: w308 -> [_]
          timing-out: [_] -> w307
          tunnel: [w321] -> w306
          tunnel: w305 -> [w320]
          stop <- w322 stop-if-true
          n191 = node-c288() -> ()  [unwired: 1 in, 1 out]
          n192 = local read "Flight Number"() -> (w334:string)
          n193 = Select(t=FALSE, s=w331, f=TRUE) -> (s? t:f=w328:bool)
          "UDP packet \nstatus" <- w328
          n194 = feedback-in #2(w334) -> ()
          n195 = feedback #2() -> (w333:string)  [unwired: 1 in]
          n196 = Not Equal?(x=w334, y=w333) -> (x != y?=w332:bool)
          n197 = flat-sequence {
            tunnel: w327 -> [w347]
            tunnel: w338 -> [w348]
            tunnel: w339 -> [w349]
            tunnel: [w349] -> w337
            tunnel: [w348] -> w336
            tunnel: [w347] -> w335
            tunnel: w332 -> [w346]
            tunnel: w326 -> [w359]
            tunnel: w337 -> [w358]
            tunnel: w336 -> [w357]
            tunnel: w335 -> [w356]
            tunnel: [w355] -> w325
            tunnel: [w354] -> w323
            tunnel: w320 -> [w353]
            frame #0 {
              n198 = feedback #3(u32 0) -> (w343:u32)
              n199 = case shown="True" w346 {
                tunnel: w343 -> [w350 _]
                tunnel: [w350 u32 0] -> w342
                frame False {
                }
                frame True {
                }
              }
              "UDP_Pack_num" <- w342
              n200 = Increment(x=w342) -> (x+1=w344:u32)
              n201 = feedback-in #3(w344) -> ()
            }
            frame #1 {
              n202 = Dequeue Element(queue=w353) -> (element=w352:string)  [unwired: 2 in, 3 out]
              n203 = UDP Write(address=w356, port or service name=w359, connection ID=w358, data in=w352, 8:w357) -> (error out=w354:errorcluster, 3:w355:refnum<k16>)  [unwired: 1 in]
            }
          }
          n204 = local read "stop"() -> (w321:bool)
          n205 = Unbundle(w323) -> ("status"=w324:bool)  [unwired: 2 out]
          n206 = node-c288() -> ()  [unwired: 1 in, 1 out]
          n207 = Compound Arithmetic op=OR(w324, w321) -> (w322:bool)
        }
        n208 = Wait (ms)(milliseconds to wait=u32 1000) -> ()  [unwired: 1 out]
        n209 = node-c288(w307) -> ()  [unwired: 1 out]
        n210 = UDP Close(connection ID=w314, 8:w312) -> (error out=→"UDP_Out_Error":errorcluster)  [unwired: 1 out]
      }
      n211 = while {
        stop <- FALSE stop-if-true
        n212 = node-c288() -> (w254:T1)  [unwired: 4 in]
        n213 = Create Network Stream Reader Endpoint(7:10 ("reader buffer size"), 9:T4 {"Message"="", "Message Data"=variant} ("Message Cluster"), 11:"/command/reader/TEi43c" ("reader url")) -> (0:w260:errorcluster, 3:w261:refnum<k21>)  [unwired: 4 in]
        n214 = timed-loop "Host->Target Command Reader" {
          shift-right: [w271] -> w258
          shift-left: w260 -> [w274]
          shift-right: [w272] -> w257
          shift-left: w261 -> [w273]
          tunnel: [TRUE] -> _
          timing: w254 -> [_]
          timing-out: [_] -> w253
          stop <- w265 stop-if-true
          # "Receive Commands from Host VI"
          n215 = node-c288() -> ()  [unwired: 1 in, 1 out]
          n216 = shared-variable-read(w273, w274) -> (w272:refnum<k21>, w267:errorcluster, w269:bool, w270:T4)  [unwired: 1 in]
          n217 = Or(x=w269, y=w267) -> (x .or. y?=w268:bool)
          n218 = case shown="False" w268 {
            selector: w268 -> [_ w300]
            tunnel: w267 -> [w282 w301]
            tunnel: [w281 w301] -> w271
            tunnel: w270 -> [w279 _]
            tunnel: [w280 w300] -> w265
            frame False {
              n219 = Unbundle By Name(w279) -> ("Message"=w278:string, "Message Data"=w277:variant)
              n220 = case shown="\"Stop\", Default" w278 {
                tunnel: w282 -> [w284 w288 w294 w299]
                tunnel: [w284 w286 w293 w298] -> w281
                tunnel: w277 -> [_ w289 w292 w297]
                tunnel: [TRUE _ _ _] -> w280
                frame "Stop", Default {
                }
                frame "Stop File Write" {
                  n221 = Variant To Data(error in=w288, type=FALSE, Variant=w289) -> (data=→"Stop File Write":bool, error out=w286:errorcluster)
                }
                frame "V6" {
                  n222 = Variant To Data(error in=w294, type=FALSE, Variant=w292) -> (data=w290:bool, error out=w293:errorcluster)
                  "V6" <- w290
                  n223 = shared-variable "NI-cRIO9022-019C2C95\\Mod6\\DO4"(w290) -> ()  [unwired: 1 in, 1 out]
                }
                frame "Flight Number" {
                  n224 = Variant To Data(error in=w299, type="", Variant=w297) -> (data=→"Flight Number":string, error out=w298:errorcluster)
                }
              }
            }
            frame True {
            }
          }
          n225 = node-c288() -> ()  [unwired: 1 in, 1 out]
        }
        n226 = node-c288(w253) -> ()  [unwired: 1 out]
        n227 = Destroy Stream Endpoint(8:w258, 11:w257) -> (0:→"error out":errorcluster)
        n228 = Wait (ms)(milliseconds to wait=u32 1000) -> ()  [unwired: 1 out]
      }
      n229 = while {
        tunnel: w48 -> [w71]
        tunnel: w49 -> [w70]
        stop <- w74 stop-if-true
        # "Must delay to avoid 100% CPU on cRIO"
        # "TCP Loop writing to SEPTIC Tank"
        n230 = TCP Open Connection(address="192.168.101.108", remote port or service name=u16 3502) -> (connection ID=w77:refnum<k5>, error out=w72:errorcluster)  [unwired: 3 in]
        n231 = case shown="No Error" w72 {
          selector: w72 -> [w82 w109]
          tunnel: w77 -> [w87 w110]
          tunnel: [w86 w110] -> w76
          tunnel: [w85 w109] -> w75
          tunnel: [w84 w108] -> w74
          tunnel: w70 -> [w81 _]
          tunnel: w71 -> [w80 _]
          frame No Error {
            n232 = node-c288() -> (w89:T1)  [unwired: 4 in]
            n233 = timed-loop {
              tunnel: w87 -> [w103]
              tunnel: w82 -> [w102]
              tunnel: [w101] -> w86
              tunnel: [w100] -> w85
              tunnel: [w90] -> w84
              shift-right: [w94] -> _
              shift-left: FALSE -> [w97]
              timing: w89 -> [_]
              timing-out: [_] -> w88
              tunnel: w81 -> [w93]
              tunnel: w80 -> [w92]
              stop <- w98 stop-if-true
              n234 = node-c288() -> ()  [unwired: 1 in, 1 out]
              n235 = Dequeue Element(queue=w93, error in (no error)=w92) -> (element=w91:string)  [unwired: 1 in, 3 out]
              n236 = Select(t=FALSE, s=w97, f=TRUE) -> (s? t:f=w94:bool)
              "TCP packet\nSend to SEPTIC" <- w94
              n237 = TCP Write(connection ID=w103, data in=w91, error in (no error)=w102) -> (connection ID out=w101:refnum<k5>, error out=w100:errorcluster)  [unwired: 1 in, 1 out]
              n238 = local read "stop"() -> (w90:bool)
              n239 = Unbundle(w100) -> ("status"=w99:bool)  [unwired: 2 out]
              n240 = node-c288() -> ()  [unwired: 1 in, 1 out]
              n241 = Compound Arithmetic op=OR(w99, w90) -> (w98:bool)
            }
            n242 = node-c288(w88) -> ()  [unwired: 1 out]
          }
          frame Error {
            n243 = local read "stop"() -> (w108:bool)
          }
        }
        n244 = TCP Close Connection(connection ID=w76, error in (no error)=w75) -> (error out=→"SEPTIC TCP Error Out":errorcluster)  [unwired: 1 in, 1 out]
        n245 = Wait (ms)(milliseconds to wait=u32 1000) -> ()  [unwired: 1 out]
      }
      n246 = while {
        tunnel: w57 -> [w113]
        tunnel: w56 -> [w112]
        stop <- w116 stop-if-true
        # "Must delay to avoid 100% CPU on cRIO"
        # "TCP Loop writing to FISH Tank"
        n247 = TCP Open Connection(address="192.168.101.110", remote port or service name=u16 3502) -> (connection ID=w119:refnum<k5>, error out=w114:errorcluster)  [unwired: 3 in]
        n248 = case shown="No Error" w114 {
          selector: w114 -> [w124 w151]
          tunnel: w119 -> [w129 w152]
          tunnel: [w128 w152] -> w118
          tunnel: [w127 w151] -> w117
          tunnel: [w126 w150] -> w116
          tunnel: w113 -> [w123 _]
          tunnel: w112 -> [w122 _]
          frame No Error {
            n249 = node-c288() -> (w131:T1)  [unwired: 4 in]
            n250 = timed-loop {
              tunnel: w129 -> [w145]
              tunnel: w124 -> [w144]
              tunnel: [w143] -> w128
              tunnel: [w142] -> w127
              tunnel: [w139] -> w126
              shift-right: [w135] -> _
              shift-left: FALSE -> [w138]
              timing: w131 -> [_]
              timing-out: [_] -> w130
              tunnel: w123 -> [w134]
              tunnel: w122 -> [w133]
              stop <- w140 stop-if-true
              n251 = node-c288() -> ()  [unwired: 1 in, 1 out]
              n252 = Dequeue Element(queue=w134, error in (no error)=w133) -> (element=w132:string)  [unwired: 1 in, 3 out]
              n253 = Select(t=FALSE, s=w138, f=TRUE) -> (s? t:f=w135:bool)
              "TCP packet\nSend to FISH" <- w135
              n254 = TCP Write(connection ID=w145, data in=w132, error in (no error)=w144) -> (connection ID out=w143:refnum<k5>, error out=w142:errorcluster)  [unwired: 1 in, 1 out]
              n255 = local read "stop"() -> (w139:bool)
              n256 = Unbundle(w142) -> ("status"=w141:bool)  [unwired: 2 out]
              n257 = node-c288() -> ()  [unwired: 1 in, 1 out]
              n258 = Compound Arithmetic op=OR(w141, w139) -> (w140:bool)
            }
            n259 = node-c288(w130) -> ()  [unwired: 1 out]
          }
          frame Error {
            n260 = local read "stop"() -> (w150:bool)
          }
        }
        n261 = TCP Close Connection(connection ID=w118, error in (no error)=w117) -> (error out=→"FISH TCP Error Out":errorcluster)  [unwired: 1 in, 1 out]
        n262 = Wait (ms)(milliseconds to wait=u32 1000) -> ()  [unwired: 1 out]
      }
      n263 = node-c288(w43) -> ()  [unwired: 1 out]
    }
    frame Error {
    }
  }
  n264 = VISA Close(VISA resource name=w22, error in (no error)=w21) -> (error out=→"Serial Visa Error":errorcluster)
